vi "Main.vi"() -> ()   [LabVIEW 2026]
doc: "This template is for the Queued Message Handler design pattern.\n\nThe Event Handling Loop generates messages based on user interface actions.\n\nThe Message Handling Loop processes messages generated by the Event Handling Loop, or by other messages. The messages are string values, so new messages can be added easily to the Message Cases case structure in the Message Handling Loop. Each message cluster can also provide an optional value for Message Data, which is a variant that can be converted to whatever message-specific data is required."
uses:
  controls/UI Data.ctl
  controls/Product.ctl
  controls/Currency.ctl
  controls/Currency Enum.ctl
  controls/Dispense Data.ctl
  support/Message Queue/Enqueue Message (Single).vi
  <vilib>/Utility/error.llb/Error Cluster From Error Code.vi
  <vilib>/ErrorRing/Error Ring.xnode
  support/Message Queue/Message Queue.lvlib
  support/User Event - Stop/User Event - Stop.lvlib
panel:
  out "Change Return":dbl
  in  "Coin Return":bool
  out "Dispensed Item":string
  out "Balance":dbl format="%_3g"
  in  "Dollar":bool
  in  "Quarter":bool
  in  "Dime":bool
  in  "Nickel":bool
  out "Chips Count":i32
  out "Chips Price":dbl
  in  "Chips":bool
  out "Cola Count":i32
  out "Cola Price":dbl
  in  "Cola":bool
  out "Candy Count":i32
  out "Candy Price":dbl
  in  "Candy":bool
  in  "Mode":bool
  out "Display":string
  in  "Exit":bool
  # "Regular"
  # "Maintenance"
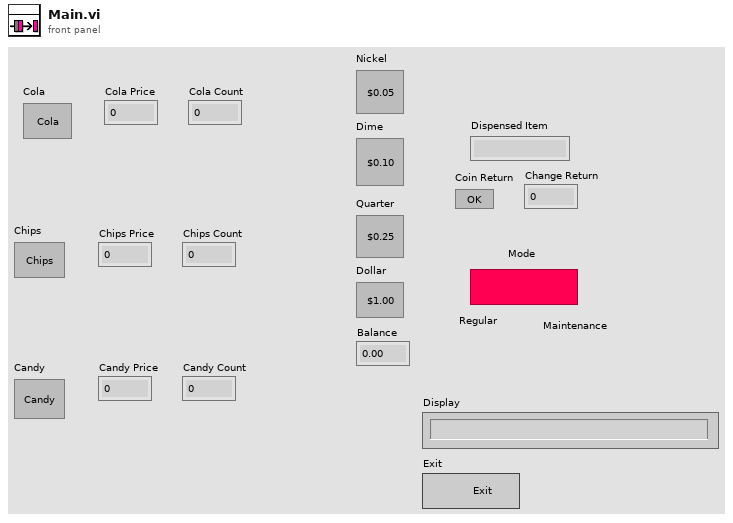
[diagram p1: front panel]
types:
  T1 = typedef "Dispense Data.ctl" = cluster{"Dispensed Item":string, "Coin Return":bool, "Change Return":dbl}
  T2 = typedef "Currency.ctl" = cluster{"Nickel":bool, "Dime":bool, "Quarter":bool, "Dollar":bool, "Balance":dbl, "Enum":T3}
  T3 = typedef "Currency Enum.ctl" = enum16{"Nickel", "Dime", "Quarter", "Dollar"}
  T4 = typedef "Product.ctl" = cluster{"Purchase Pressed":bool, "Price":dbl, "Count":i32}
  T5 = typedef "UI Data.ctl" = cluster{"Boolean <Replace Me>":bool, "String <Replace Me>":string, "Numeric <Replace Me>":dbl, "Do Something Ref":refnum<vi>, "Do Something Else Ref":refnum<vi>, "Data Display Ref":refnum<vi>, "Exit Button Ref":refnum<vi>}
  T6 = typedef "Message Queue.lvlib/All Message Queues.ctl" = cluster{"UI":refnum<queue>}
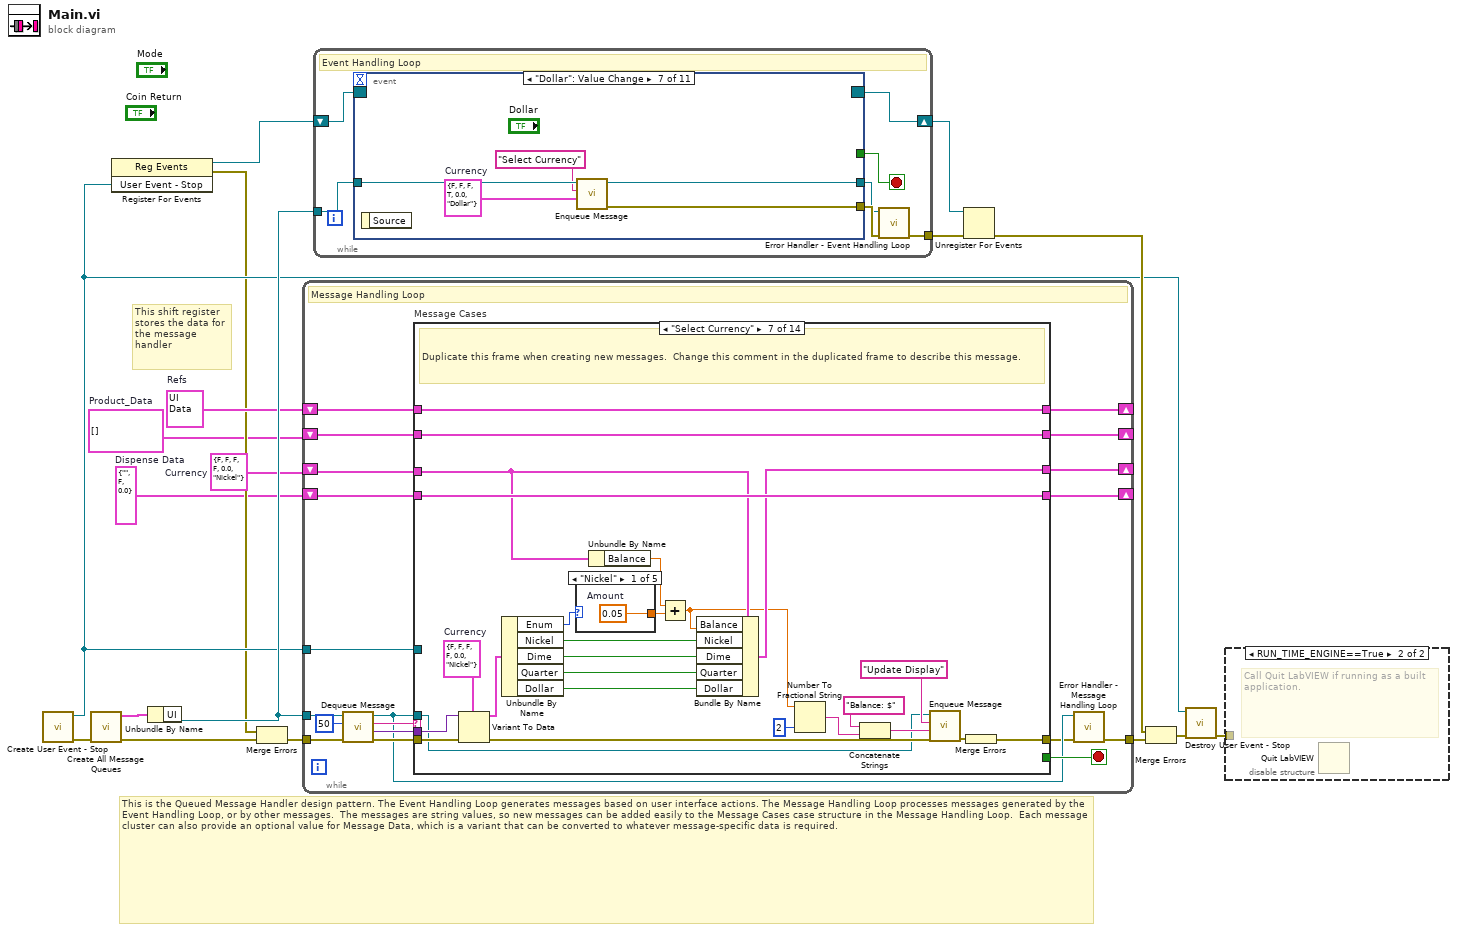
[diagram p0: block diagram]
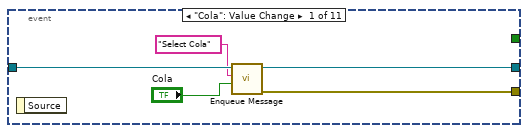
[diagram p3: hidden frame]
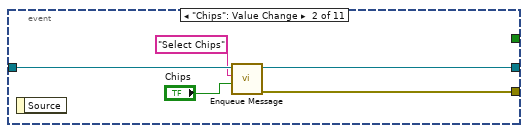
[diagram p4: hidden frame]
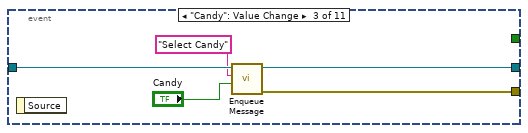
[diagram p5: hidden frame]
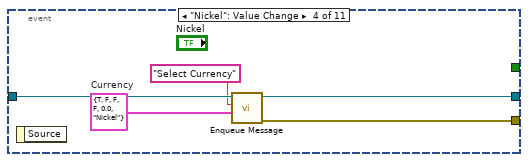
[diagram p6: hidden frame]
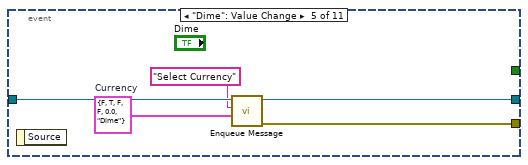
[diagram p7: hidden frame]
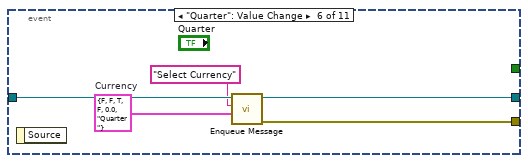
[diagram p8: hidden frame]
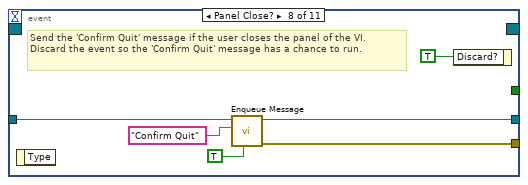
[diagram p9: hidden frame]
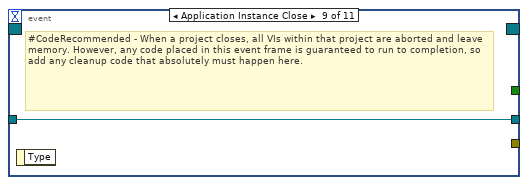
[diagram p10: hidden frame]
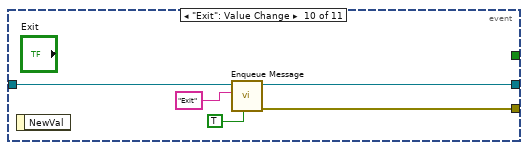
[diagram p11: hidden frame]
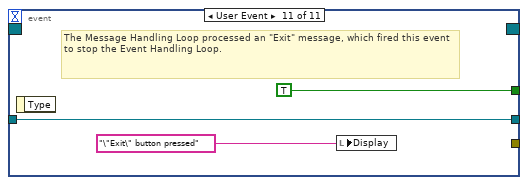
[diagram p12: hidden frame]
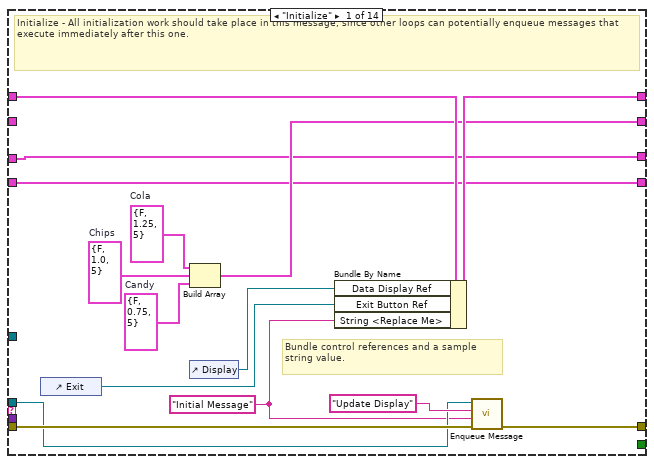
[diagram p13: hidden frame]
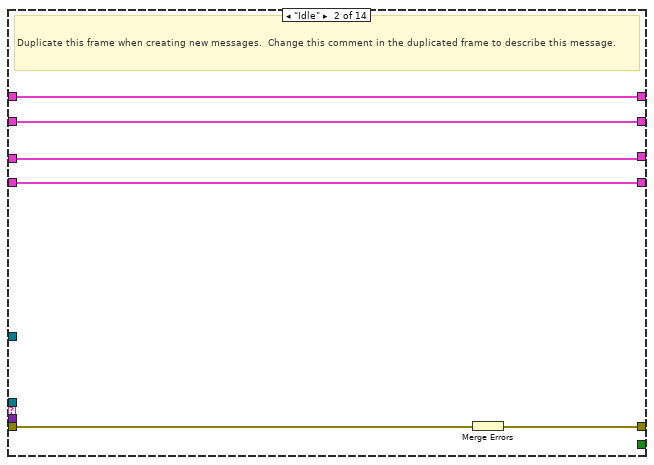
[diagram p14: hidden frame]
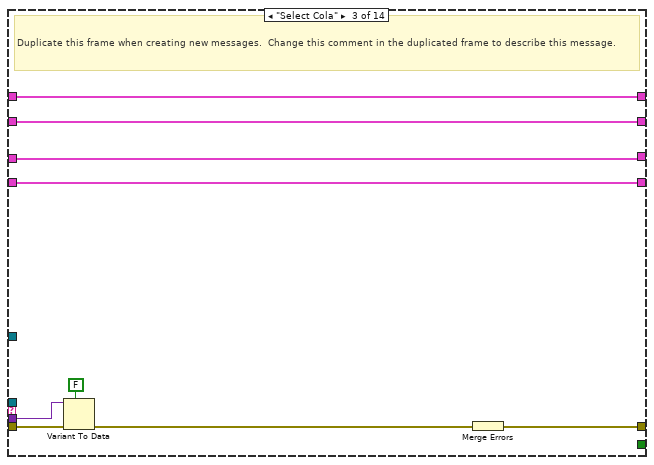
[diagram p15: hidden frame]
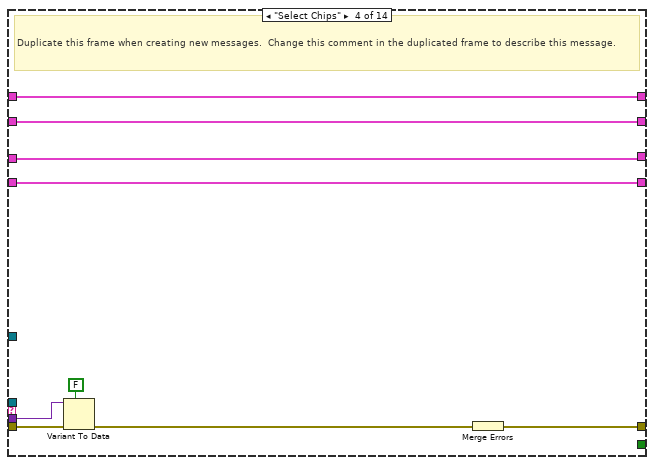
[diagram p16: hidden frame]
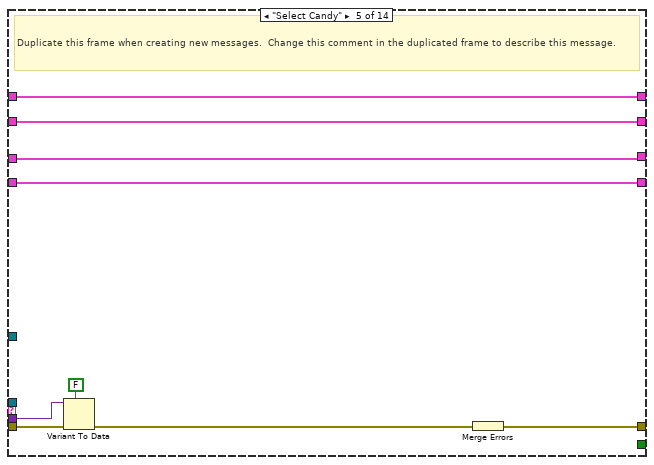
[diagram p17: hidden frame]
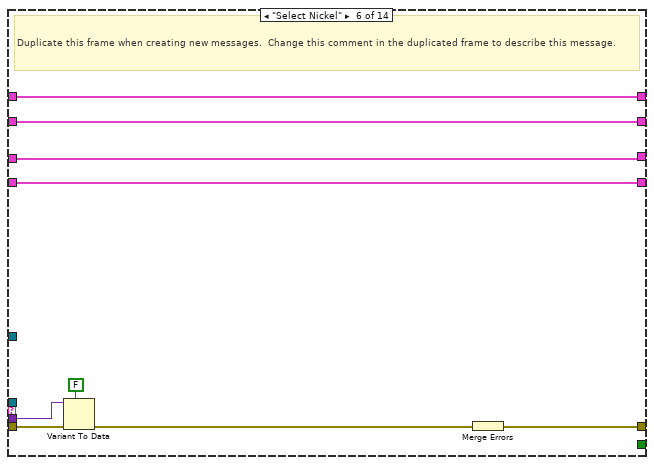
[diagram p18: hidden frame]
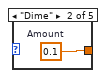
[diagram p19: hidden frame]
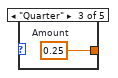
[diagram p20: hidden frame]
diagram:
  w1 = T1 {"Dispensed Item"="", "Coin Return"=FALSE, "Change Return"=0.0}  # Dispense Data
  w2 = T2 {"Nickel"=FALSE, "Dime"=FALSE, "Quarter"=FALSE, "Dollar"=FALSE, "Balance"=0.0, "Enum"=enum."Nickel"}  # Currency
  w3 = T4[] []  # Product_Data
  w10 = T5 {"Boolean <Replace Me>"=FALSE, "String <Replace Me>"="", "Numeric <Replace Me>"=0.0, "Do Something Ref"=refnum, "Do Something Else Ref"=refnum, "Data Display Ref"=refnum, "Exit Button Ref"=refnum}  # Refs
  # "This is the Queued Message Handler design pattern. The Event Handling Loop generates messages based on user interface actions. The Message Handling Loop processes messages generated by the Event Handling Loop, or by other messages.  The messages are string values, so new messages can be added easily to the Message Cases case structure in the Message Handling Loop.  Each message cluster can also provide an optional value for Message Data, which is a variant that can be converted to whatever message-specific data is required."
  # "This shift register stores the data for the message handler"
  n1 = call "Create User Event - Stop.vi"() -> ("error out"=w14:errorcluster, "User Event - Stop"=w6:refnum<user-event>)  [unwired: 10 in]
  n2 = call "Create All Message Queues.vi"("error in (no error)"=w14) -> ("error out"=w18:errorcluster, "Message Queues out"=w17:T6)  [unwired: 9 in]
  n3 = register-events(w6) -> (reference out=w7:refnum<event-registration>, error out=w4:errorcluster)  [unwired: 2 in]
  n4 = Unbundle By Name(w17) -> ("UI"=w15:refnum<queue>)
  n5 = Merge Errors(w4, w18) -> (w5:errorcluster)
  n6 = while {
    tunnel: w15 -> [w29]
    shift-right: [w36] -> _
    shift-left: w10 -> [w37]
    tunnel: w6 -> [w34]
    tunnel: w5 -> [w33]
    tunnel: [w27] -> w16
    shift-right: [w24] -> _
    shift-left: w3 -> [w23]
    shift-right: [w21] -> _
    shift-left: w2 -> [w22]
    shift-right: [w19] -> _
    shift-left: w1 -> [w20]
    stop <- w35 stop-if-true
    # "Message Handling Loop"
    n7 = call "Dequeue Message.vi"("error in (no error)"=w33, "timeout in ms (-1)"=50, "Message Queue"=w29) -> ("error out"=w32:errorcluster, "Message Data"=w30:variant, "Message"=w31:string, "dup Message Queue"=w28:refnum<queue>)  [unwired: 5 in]
    n8 = case "Message Cases" shown="\"Select Currency\"" w31 {
      selector: w31 -> [_ _ _ _ _ _ _ _ _ _ _ _ _ w195]
      tunnel: w28 -> [w45 _ _ _ _ _ w97 _ _ w161 _ _ w191 _]
      tunnel: w32 -> [w51 w58 w62 w71 w80 w89 w116 w143 w155 w165 w171 w177 w184 _]
      tunnel: [w52 w56 w66 w75 w84 w93 w119 w144 w149 w163 w169 w175 w187 w196] -> w26
      tunnel: w37 -> [w50 w57 w67 w76 w85 w94 w120 w145 w154 w164 w170 w176 w190 w197]
      tunnel: [w49 w57 w67 w76 w85 w94 w120 w145 w154 w164 w170 w176 w190 w197] -> w36
      tunnel: [_ _ _ _ _ _ _ _ _ _ _ _ TRUE _] -> w35
      tunnel: w30 -> [_ _ w61 w70 w79 w88 w115 w142 w153 _ _ _ w181 _]
      tunnel: w34 -> [_ _ _ _ _ _ _ _ _ _ _ _ w186 _]
      tunnel: [w43 w55 w65 w74 w83 w92 w118 w137 w148 w158 w168 w174 w180 w194] -> w24
      tunnel: w23 -> [_ w55 w65 w74 w83 w92 w118 w137 w148 w158 w168 w174 w180 w194]
      tunnel: w22 -> [w39 w54 w64 w73 w82 w91 w103 w127 w147 w157 w167 w173 w179 w193]
      tunnel: [w39 w54 w64 w73 w82 w91 w108 w127 w147 w157 w167 w173 w179 w193] -> w21
      tunnel: w20 -> [w38 w53 w63 w72 w81 w90 w117 w138 w146 w156 w166 w172 w178 w192]
      tunnel: [w38 w53 w63 w72 w81 w90 w117 w138 w146 w156 w166 w172 w178 w192] -> w19
      frame "Initialize" {
        w40 = T4 {"Purchase Pressed"=FALSE, "Price"=0.75, "Count"=5}  # Candy
        w41 = T4 {"Purchase Pressed"=FALSE, "Price"=1.0, "Count"=5}  # Chips
        w42 = T4 {"Purchase Pressed"=FALSE, "Price"=1.25, "Count"=5}  # Cola
        w44 = "Initial Message" ("Initial Message")
        # "Bundle control references and a sample string value."
        # "Initialize - All initialization work should take place in this message, since other loops can potentially enqueue messages that execute immediately after this one."
        n9 = control-ref of="Exit"() -> (w47:refnum<vi>)
        n10 = Build Array(w42, w41, w40) -> (w43:T4[])
        n11 = control-ref of="Display"() -> (w48:refnum<vi>)
        n12 = Bundle By Name(cluster=w50, "Data Display Ref"=w48, "Exit Button Ref"=w47, "String <Replace Me>"=w44) -> (w49:T5)
        n13 = call-poly "Enqueue Message.vi"("error in (no error)"=w51, "Message Data"=w44, "Message"="Update Display", "Message Queue"=w45) -> ("error out"=w52:errorcluster)  [unwired: 6 in, 1 out]
      }
      frame "Idle" {
        # "Duplicate this frame when creating new messages.  Change this comment in the duplicated frame to describe this message."
        n14 = Merge Errors(w58) -> (w56:errorcluster)
      }
      frame "Select Cola" {
        # "Duplicate this frame when creating new messages.  Change this comment in the duplicated frame to describe this message."
        n15 = Variant To Data(error in=w62, type=FALSE, Variant=w61) -> (error out=w59:errorcluster)  [unwired: 1 out]
        n16 = Merge Errors(w59) -> (w66:errorcluster)
      }
      frame "Select Chips" {
        # "Duplicate this frame when creating new messages.  Change this comment in the duplicated frame to describe this message."
        n17 = Variant To Data(error in=w71, type=FALSE, Variant=w70) -> (error out=w68:errorcluster)  [unwired: 1 out]
        n18 = Merge Errors(w68) -> (w75:errorcluster)
      }
      frame "Select Candy" {
        # "Duplicate this frame when creating new messages.  Change this comment in the duplicated frame to describe this message."
        n19 = Variant To Data(error in=w80, type=FALSE, Variant=w79) -> (error out=w77:errorcluster)  [unwired: 1 out]
        n20 = Merge Errors(w77) -> (w84:errorcluster)
      }
      frame "Select Nickel" {
        # "Duplicate this frame when creating new messages.  Change this comment in the duplicated frame to describe this message."
        n21 = Variant To Data(error in=w89, type=FALSE, Variant=w88) -> (error out=w86:errorcluster)  [unwired: 1 out]
        n22 = Merge Errors(w86) -> (w93:errorcluster)
      }
      frame "Select Currency" {
        w114 = T2 {"Nickel"=FALSE, "Dime"=FALSE, "Quarter"=FALSE, "Dollar"=FALSE, "Balance"=0.0, "Enum"=enum."Nickel"}  # Currency
        # "Duplicate this frame when creating new messages.  Change this comment in the duplicated frame to describe this message."
        n23 = Variant To Data(error in=w116, type=w114, Variant=w115) -> (data=w113:T2, error out=w107:errorcluster)
        n24 = Unbundle By Name(w113) -> ("Enum"=w104:T3, "Nickel"=w112:bool, "Dime"=w111:bool, "Quarter"=w110:bool, "Dollar"=w109:bool)
        n25 = case shown="\"Nickel\"" w104 {
          tunnel: [w121 w122 w123 w124 0.0 ("Amount")] -> w101
          frame "Nickel" {
            w121 = 0.05  # Amount
          }
          frame "Dime" {
            w122 = 0.1  # Amount
          }
          frame "Quarter" {
            w123 = 0.25  # Amount
          }
          frame "Dollar" {
            w124 = 1.0  # Amount
          }
          frame Default {
          }
        }
        n26 = Unbundle By Name(w103) -> ("Balance"=w102:dbl)
        n27 = Add(x=w102, y=w101) -> (x+y=w96:dbl)
        n28 = Bundle By Name(cluster=w103, "Balance"=w96, "Nickel"=w112, "Dime"=w111, "Quarter"=w110, "Dollar"=w109) -> (w108:T2)
        n29 = Number To Fractional String(number=w96, precision (6)=i16 2) -> (F-format string=w99:string)  [unwired: 2 in]
        n30 = Concatenate Strings("Balance: $" ("Message"), w99) -> (w98:string)
        n31 = call-poly "Enqueue Message.vi"("error in (no error)"=w107, "Message Data"=w98, "Message"="Update Display", "Message Queue"=w97) -> ("error out"=w106:errorcluster)  [unwired: 6 in, 1 out]
        n32 = Merge Errors(w106) -> (w119:errorcluster)
      }
      frame "Update Display" {
        # "Update Display - Convert the message data to a string to display in the Data Display indicator."
        n33 = Index Array(array=w137) -> (element #1=w136:T4, element #2=w131:T4, element #3=w130:T4)  [unwired: 3 in]
        n34 = Variant To Data(error in=w143, type="", Variant=w142) -> (data=→"Display":string, error out=w140:errorcluster)
        n35 = Unbundle By Name(w127) -> ("Balance"=→"Balance":dbl)
        n36 = Unbundle By Name(w130) -> ("Price"=→"Candy Price":dbl, "Count"=→"Candy Count":i32)
        n37 = Unbundle By Name(w131) -> ("Price"=→"Chips Price":dbl, "Count"=→"Chips Count":i32)
        n38 = Unbundle By Name(w136) -> ("Price"=→"Cola Price":dbl, "Count"=→"Cola Count":i32)
        n39 = Merge Errors(w140) -> (w144:errorcluster)
      }
      frame "Error" {
        # "#CodeRecommended - If you ever change the name of this \"Error\" message, you'll need to update the name in the Check Loop Error.vi as well."
        # "#CodeRecommended - Consider creating a system for logging errors in some way. These errors are for notification purposes only. Handling of specific errors should be performed in the message frames that generated the error."
        # "Error - Display an error dialog. This message is sent by the \"Error Handler\" VIs at the end of other loops in this application."
        n40 = Variant To Data(error in=w155, type=errorcluster {"status"=FALSE, "code"=0, "source"=""} ("error constant"), Variant=w153) -> (data=w151:errorcluster, error out=w150:errorcluster)
        n41 = call <vilib>:"Simple Error Handler.vi"("error in (no error)"=w151) -> ()  [unwired: 4 in, 5 out]
        n42 = Merge Errors(w150) -> (w149:errorcluster)
      }
      frame "Confirm Quit" {
        # "#CodeNeeded - If you want to provide an \"Are you sure\" dialog (or some other notification) before the application exits, place that code here. This message is typically sent from a Panel Close? event."
        # "Confirm Quit - Message that can confirm whether or not the user wants to exit the application."
        n43 = call-poly "Enqueue Message.vi"("Priority Message? (F)"=TRUE, "error in (no error)"=w165, "Message"="Exit", "Message Queue"=w161) -> ("error out"=w162:errorcluster)  [unwired: 6 in, 1 out]
        n44 = Merge Errors(w162) -> (w163:errorcluster)
      }
      frame "---Copy This Frame---" {
        # "Duplicate this frame when creating new messages.  Change this comment in the duplicated frame to describe this message."
        n45 = Merge Errors(w171) -> (w169:errorcluster)
      }
      frame "Timeout" {
        # "Duplicate this frame when creating new messages.  Change this comment in the duplicated frame to describe this message."
        n46 = Merge Errors(w177) -> (w175:errorcluster)
      }
      frame "Exit" {
        # "Stop the VI"
        # "Release the message queue reference"
        # "#CodeNeeded - Add any required cleanup code here. Note that if 'Exit' was called as a result of an error, an error dialog will be displayed. Add any custom error handling for an 'Exit' condition here as well."
        # "Exit - Exit the application."
        n47 = Variant To Data(type=errorcluster {"status"=FALSE, "code"=0, "source"=""} ("error constant"), Variant=w181) -> (data=w182:errorcluster)  [unwired: 1 in, 1 out]
        n48 = call <vilib>:"Simple Error Handler.vi"("error in (no error)"=w182) -> ()  [unwired: 4 in, 5 out]
        n49 = call "Fire User Event - Stop.vi"("User Event - Stop"=w186) -> ("error out"=w185:errorcluster)  [unwired: 10 in]
        n50 = Release Queue(queue=w191, error in (no error)=w184) -> (error out=w188:errorcluster)  [unwired: 1 in, 2 out]
        n51 = Merge Errors(w185, w188) -> (w187:errorcluster)
      }
      frame Default {
        # "'Default' case only runs if there is a message that isn't defined in any of the other cases.  Output a programming error."
        n52 = xnode "Error Ring"("parameter 0"=w195) -> ("error out"=w196:errorcluster)
      }
    }
    n53 = call "Error Handler - Message Handling Loop.vi"("error in (no error)"=w26, "Message Queue"=w28) -> ("dup error in"=w27:errorcluster)  [unwired: 8 in, 1 out]
  }
  n54 = while {
    tunnel: w15 -> [w211]
    shift-right: [w209] -> w11
    shift-left: w7 -> [w210]
    tunnel: [w205] -> w8
    stop <- w207 stop-if-true
    # "Event Handling Loop"
    n55 = event shown="[6] \"Dollar\": Value Change" {
      selector: w210 -> [_ _ _ _ _ _ _ _ _ _ _]
      dyn-events: [_ _ _ _ _ _ _ _ _ _ _] -> w209
      timeout: _ -> [_ _ _ _ _ _ _ _ _ _ _]
      tunnel: [_ _ _ _ _ _ _ _ _ _ TRUE ("Discard?")] -> w207
      tunnel: w211 -> [w216 w221 w226 w231 w236 w241 w246 w251 w253 w258 w261]
      tunnel: [w215 w220 w225 w230 w235 w240 w245 w250 _ w257 _] -> w208
      tunnel: [w214 w219 w224 w229 w234 w239 w244 w249 w253 w256 w261] -> w206
      event "Cola": Value Change {
        n56 = event-data() -> ()  [unwired: 1 in, 1 out]
        n57 = call-poly "Enqueue Message.vi"("Message Data"="Cola", "Message"="Select Cola", "Message Queue"=w216) -> ("error out"=w215:errorcluster, "dup Message Queue"=w214:refnum<queue>)  [unwired: 7 in]
      }
      event "Chips": Value Change {
        n58 = event-data() -> ()  [unwired: 1 in, 1 out]
        n59 = call-poly "Enqueue Message.vi"("Message Data"="Chips", "Message"="Select Chips", "Message Queue"=w221) -> ("error out"=w220:errorcluster, "dup Message Queue"=w219:refnum<queue>)  [unwired: 7 in]
      }
      event "Candy": Value Change {
        n60 = event-data() -> ()  [unwired: 1 in, 1 out]
        n61 = call-poly "Enqueue Message.vi"("Message Data"="Candy", "Message"="Select Candy", "Message Queue"=w226) -> ("error out"=w225:errorcluster, "dup Message Queue"=w224:refnum<queue>)  [unwired: 7 in]
      }
      event "Nickel": Value Change {
        w227 = T2 {"Nickel"=TRUE, "Dime"=FALSE, "Quarter"=FALSE, "Dollar"=FALSE, "Balance"=0.0, "Enum"=enum."Nickel"}  # Currency
        n62 = event-data() -> ()  [unwired: 1 in, 1 out]
        n63 = call-poly "Enqueue Message.vi"("Message Data"=w227, "Message"="Select Currency", "Message Queue"=w231) -> ("error out"=w230:errorcluster, "dup Message Queue"=w229:refnum<queue>)  [unwired: 7 in]
      }
      event "Dime": Value Change {
        w232 = T2 {"Nickel"=FALSE, "Dime"=TRUE, "Quarter"=FALSE, "Dollar"=FALSE, "Balance"=0.0, "Enum"=enum."Dime"}  # Currency
        n64 = event-data() -> ()  [unwired: 1 in, 1 out]
        n65 = call-poly "Enqueue Message.vi"("Message Data"=w232, "Message"="Select Currency", "Message Queue"=w236) -> ("error out"=w235:errorcluster, "dup Message Queue"=w234:refnum<queue>)  [unwired: 7 in]
      }
      event "Quarter": Value Change {
        w237 = T2 {"Nickel"=FALSE, "Dime"=FALSE, "Quarter"=TRUE, "Dollar"=FALSE, "Balance"=0.0, "Enum"=enum."Quarter"}  # Currency
        n66 = event-data() -> ()  [unwired: 1 in, 1 out]
        n67 = call-poly "Enqueue Message.vi"("Message Data"=w237, "Message"="Select Currency", "Message Queue"=w241) -> ("error out"=w240:errorcluster, "dup Message Queue"=w239:refnum<queue>)  [unwired: 7 in]
      }
      event "Dollar": Value Change {
        w242 = T2 {"Nickel"=FALSE, "Dime"=FALSE, "Quarter"=FALSE, "Dollar"=TRUE, "Balance"=0.0, "Enum"=enum."Dollar"}  # Currency
        n68 = event-data() -> ()  [unwired: 1 in, 1 out]
        n69 = call-poly "Enqueue Message.vi"("Message Data"=w242, "Message"="Select Currency", "Message Queue"=w246) -> ("error out"=w245:errorcluster, "dup Message Queue"=w244:refnum<queue>)  [unwired: 7 in]
      }
      event Panel Close? {
        # "Send the 'Confirm Quit' message if the user closes the panel of the VI. Discard the event so the 'Confirm Quit' message has a chance to run."
        n70 = event-data() -> ()  [unwired: 1 in, 1 out]
        n71 = call-poly "Enqueue Message.vi"("Priority Message? (F)"=TRUE, "Message"="Confirm Quit", "Message Queue"=w251) -> ("error out"=w250:errorcluster, "dup Message Queue"=w249:refnum<queue>)  [unwired: 7 in]
        n72 = event-data("Discard?"=TRUE) -> ()  [unwired: 1 in, 1 out]
      }
      event Application Instance Close {
        # "#CodeRecommended - When a project closes, all VIs within that project are aborted and leave memory. However, any code placed in this event frame is guaranteed to run to completion, so add any cleanup code that absolutely must happen here."
        n73 = event-data() -> ()  [unwired: 1 in, 1 out]
      }
      event "Exit": Value Change {
        n74 = event-data() -> ()  [unwired: 1 in, 1 out]
        n75 = call-poly "Enqueue Message.vi"("Priority Message? (F)"=TRUE, "Message"="Exit", "Message Queue"=w258) -> ("error out"=w257:errorcluster, "dup Message Queue"=w256:refnum<queue>)  [unwired: 7 in]
      }
      event User Event {
        # "The Message Handling Loop processed an \"Exit\" message, which fired this event to stop the Event Handling Loop."
        n76 = event-data() -> ()  [unwired: 1 in, 1 out]
        n77 = local write "Display"("\"Exit\" button pressed" ("VI Stopped")) -> ()
      }
    }
    n78 = call "Error Handler - Event Handling Loop.vi"("error in (no error)"=w208, "Message Queue"=w206) -> ("dup error in"=w205:errorcluster)  [unwired: 8 in, 1 out]
  }
  n79 = Unregister For Events(event registration refnum=w11, error in=w8) -> (error out=w12:errorcluster)
  n80 = Merge Errors(w12, w16) -> (w13:errorcluster)
  n81 = call "Destroy User Event - Stop.vi"("error in (no error)"=w13, "User Event - Stop"=w6) -> ("error out"=w9:errorcluster)  [unwired: 9 in]
  n82 = disable-structure shown="RUN_TIME_ENGINE==True" {
    disable-tunnel: w9 -> [_ _]
    frame condition #0 (active) {
    }
    frame condition #1 {
      # "Call Quit LabVIEW if running as a built application."
      n83 = Quit LabVIEW() -> ()  [unwired: 1 in]
    }
  }
